vi "GetDefaultParams.vi"(8 "error in (no error)":errorcluster, 10 "ConfigFilePath":path, 11 "BaseWfrmPlugin in":refnum<class "BaseWfrmPlugin.lvclass">) -> (0 "error out":errorcluster, 3 "BaseWfrmPlugin out":refnum<class "BaseWfrmPlugin.lvclass">)   [LabVIEW 2014, in "WfrmPlugins.lvlib" / "BaseWfrmPlugin.lvclass"]
uses:
  BaseWfrmPlugin.lvclass
  TypeDefs/clWfrmParams.ctl
  TypeDefs/WfrmConfig.ctl
  BaseWfrmPlugin.lvclass/BaseWfrmPlugin.ctl
  Accessors/Write clWfrmParams.vi
  Accessors/Write StartTime.vi
  Accessors/Write EndTime.vi
  Accessors/Write SettlingTime.vi
  <vilib>/Utility/config.llb/NI_LVConfig.lvlib
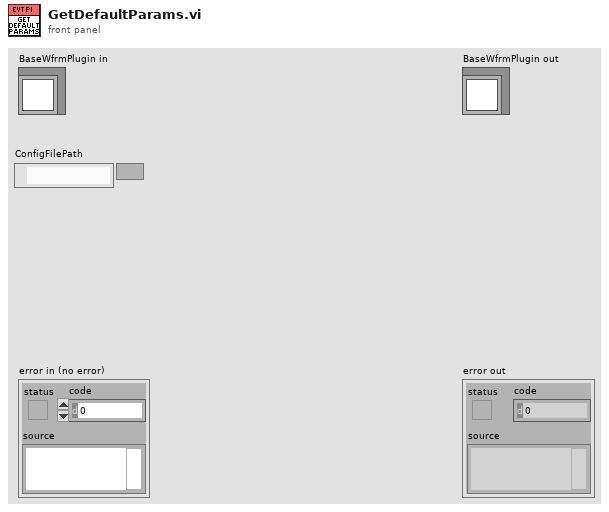
[diagram p1: front panel]
types:
  T1 = typedef "WfrmPlugins.lvlib/BaseWfrmPlugin.lvclass/WfrmConfig.ctl" = cluster{"T0(UTC)":dbl, "F0":dbl, "Fs":i32, "FSamp":u32}
  T2 = typedef "WfrmPlugins.lvlib/BaseWfrmPlugin.lvclass/clWfrmParams.ctl" = cluster{"RowHdrs":string[], "ColHdrs":string[], "DefaultParams":string[][]}
  T3 = typedef "NI_LVConfig.lvlib/Config Data RefNum.ctl" = refnum<k1>
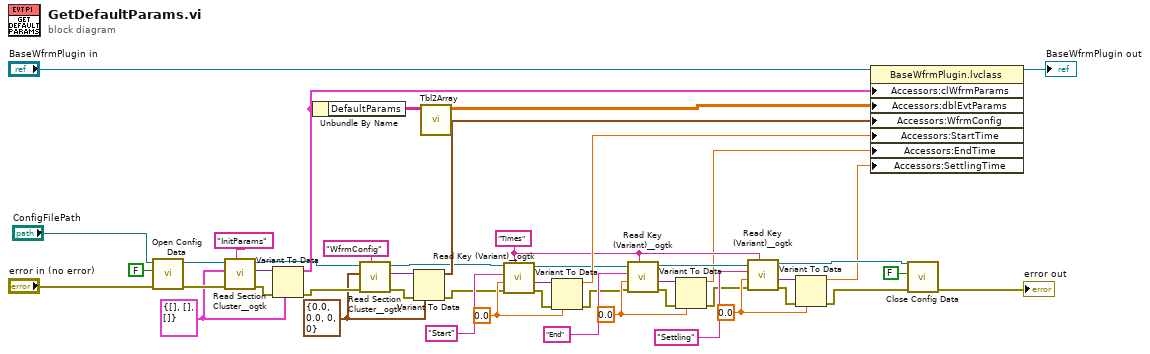
[diagram p0: block diagram]
diagram:
  w13 = 0.0 ("SettlingTime")
  w18 = 0.0 ("SettlingTime")
  w21 = 0.0 ("SettlingTime")
  w7 = "Times" ("section")
  w26 = T1 {"T0(UTC)"=0.0, "F0"=0.0, "Fs"=0, "FSamp"=0} ("WfrmConfig")
  w38 = T2 {"RowHdrs"=[], "ColHdrs"=[], "DefaultParams"=[]} ("clWfrmParams")
  n1 = call <vilib>:"Open Config Data.vi"("error in (no error)"="error in (no error)", "create file if necessary (T)"=FALSE, "configuration file path"="ConfigFilePath") -> ("error out"=w43:errorcluster, "refnum"=w42:T3)  [unwired: 6 in, 1 out]
  n2 = call <userlib>:"Read Section Cluster__ogtk.vi"("section (optional)"="InitParams", "error in (no error)"=w43, "Section Formatted Cluster Type"=w38, "refnum"=w42) -> ("error out"=w39:errorcluster, "Section Formatted Cluster"=w40:variant, "dup refnum"=w29:T3)  [unwired: 3 in, 2 out]
  n3 = Variant To Data(error in=w39, type=w38, Variant=w40) -> (data=w36:T2, error out=w31:errorcluster)
  n4 = Unbundle By Name(w36) -> ("DefaultParams"=w33:string[][])
  n5 = call <userlib>:"Read Section Cluster__ogtk.vi"("section (optional)"="WfrmConfig", "error in (no error)"=w31, "Section Formatted Cluster Type"=w26, "refnum"=w29) -> ("error out"=w30:errorcluster, "Section Formatted Cluster"=w28:variant, "dup refnum"=w24:T3)  [unwired: 3 in, 2 out]
  n6 = Variant To Data(error in=w30, type=w26, Variant=w28) -> (data=w25:T1, error out=w6:errorcluster)
  n7 = call "Tbl2Array.vi"("strTable"=w33) -> ("dblArray"=w32:dbl[][])  [unwired: 10 in]
  n8 = call <userlib>:"Read Key (Variant)__ogtk.vi"("section"=w7, "error in (no error)"=w6, "type"=w21, "key (optional)"="Start", "refnum"=w24) -> ("error out"=w23:errorcluster, "key-value"=w22:variant, "refnum out"=w5:T3)  [unwired: 3 in, 1 out]
  n9 = Variant To Data(error in=w23, type=w21, Variant=w22) -> (data=w20:dbl, error out=w10:errorcluster)
  n10 = call <userlib>:"Read Key (Variant)__ogtk.vi"("section"=w7, "error in (no error)"=w10, "type"=w18, "key (optional)"="End", "refnum"=w5) -> ("error out"=w16:errorcluster, "key-value"=w17:variant, "refnum out"=w4:T3)  [unwired: 3 in, 1 out]
  n11 = Variant To Data(error in=w16, type=w18, Variant=w17) -> (data=w2:dbl, error out=w9:errorcluster)
  n12 = call <userlib>:"Read Key (Variant)__ogtk.vi"("section"=w7, "error in (no error)"=w9, "type"=w13, "key (optional)"="Settling", "refnum"=w4) -> ("error out"=w15:errorcluster, "key-value"=w14:variant, "refnum out"=w3:T3)  [unwired: 3 in, 1 out]
  n13 = Variant To Data(error in=w15, type=w13, Variant=w14) -> (data=w1:dbl, error out=w8:errorcluster)
  n14 = property class="BaseWfrmPlugin.lvclass"(reference="BaseWfrmPlugin in", "Accessors:clWfrmParams"=w36, "Accessors:dblEvtParams"=w32, "Accessors:WfrmConfig"=w25, "Accessors:StartTime"=w20, "Accessors:EndTime"=w2, "Accessors:SettlingTime"=w1) -> (reference out=→"BaseWfrmPlugin out":refnum<class "BaseWfrmPlugin.lvclass">)  [unwired: 1 in, 1 out]
  n15 = call <vilib>:"Close Config Data.vi"("error in (no error)"=w8, "write file if changed (T)"=FALSE, "refnum"=w3) -> ("error out"=→"error out":errorcluster)  [unwired: 7 in, 1 out]
